vi "Command (write) - DL.vi"(7 "timeout ms (100)":i32=100, 8 "error in (no error)":errorcluster, 9 "Parameter":string, 10 "IP":string, 11 "connection ID in":refnum<k16>) -> (0 "error out":errorcluster, 3 "connection ID out":refnum<k16>)   [LabVIEW 2016, in "SMD-7615.lvlib" / "eSCL.lvlib"]
doc: "DL - Define Limits (StepSERVO and SV200 drives)\nCW and CCW end-of-travel limits are available on all drives and can be used to define the boundaries of\nacceptable motion in a motor/drive system. If one of these inputs is activated while defined as an end-of-travel limit, motor rotation will stop in that direction, and an alarm code will show at the drive’s status LEDs. When defining these inputs as end-of-travel limits, individual or both inputs can be defined as either active low, active high, or not used. See below for details.\n\nDL1: End-of-travel limit occurs when an input is closed (energized). Motion stops automatically at rate defined by AM command.\nDL2: End-of-travel limit occurs when an input is open (de-energized). Motion stops automatically at rated\ndefined by AM command.\nDL3: Inputs are not used as end-of-travel limit inputs and can be used as a general purpose inputs. In the case of ST-S and STM drives, DL will be automatically set to 3 if CM is set to 7, 11, 12, 13, 14, 15, 16, 17, or 18, or if JE is executed after the DL command is set.\nDL7: individually set end-of-travel in CW direction when CW Limit inputs is closed(energized).\nDL8: individually set end-of-travel in CW direction when CW Limit inputs is open (de-energized).\nDL9: individually set end-of-travel in CCW direction when CCW Limit inputs is closed(energized).\nDL10: individually set end-of-travel in CCW direction when CCW Limit inputs is open (de-energized).\nDL11~13, DL17~20: Swap the CW input and CCW input definition as above setting."
uses:
  eSCL.lvlib
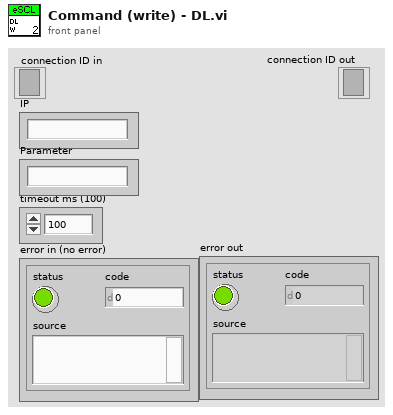
[diagram p1: front panel]
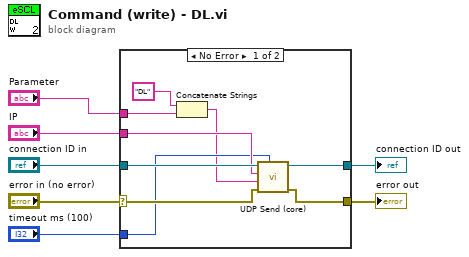
[diagram p0: block diagram]
diagram:
  n1 = case shown="No Error" "error in (no error)" {
    selector: "error in (no error)" -> [w16 w17]
    tunnel: "connection ID in" -> [w15 w18]
    tunnel: [w10 w18] -> w5
    tunnel: [w9 w17] -> w4
    tunnel: "IP" -> [w14 _]
    tunnel: "timeout ms (100)" -> [w13 _]
    tunnel: "Parameter" -> [w11 _]
    frame No Error {
      n2 = Concatenate Strings("DL" ("Data"), w11) -> (w8:string)
      n3 = call "UDP Send (core).vi"("timeout ms (100)"=w13, "error in (no error)"=w16, "Data"=w8, "IP"=w14, "connection ID in"=w15) -> ("error out"=w9:errorcluster, "connection ID out"=w10:refnum<k16>)  [unwired: 5 in]
    }
    frame Error {
    }
  }
  "connection ID out" <- w5
  "error out" <- w4
